vi "User Event Driver.vi"(11 "error in":errorcluster, 13 "LV2 Operation":T1) -> (4 "Stop":refnum<user-event>, 15 "error out":errorcluster)   [LabVIEW 2021, in "Game of Life.lvlib" / "User Event.lvlib"]
uses:
  User Event.lvlib
  controls/User Event Operations.ctl
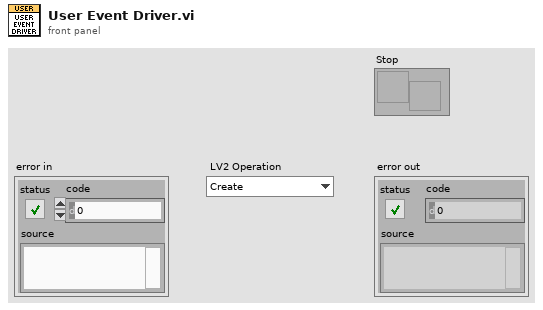
[diagram p1: front panel]
types:
  T1 = typedef "Game of Life.lvlib/User Event.lvlib/User Event Operations.ctl" = enum16{"Create", "Destroy", "Get Reference", "Generate"}
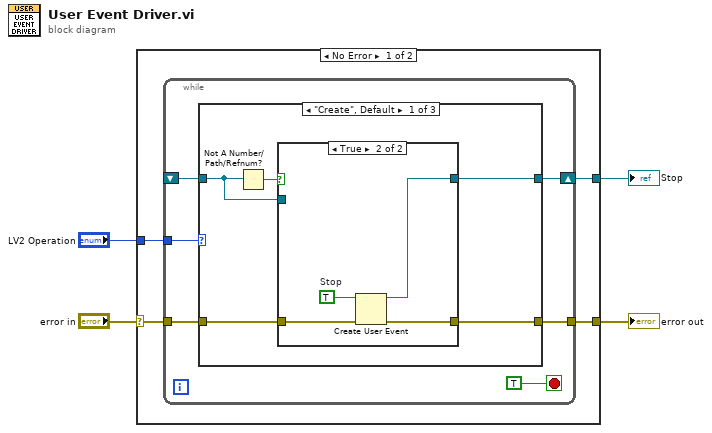
[diagram p0: block diagram]
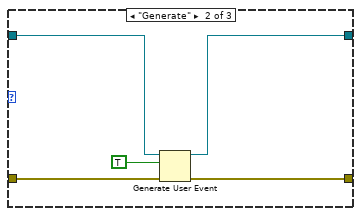
[diagram p3: hidden frame]
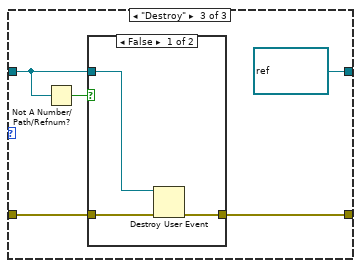
[diagram p4: hidden frame]
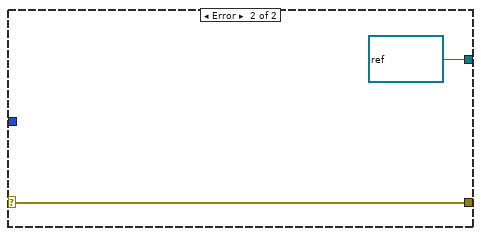
[diagram p6: hidden frame]
diagram:
  n1 = case shown="No Error" "error in" {
    selector: "error in" -> [w8 w41]
    tunnel: [w7 w41] -> w3
    tunnel: "LV2 Operation" -> [w6 _]
    tunnel: [w5 refnum<user-event> refnum ("Stop")] -> w1
    frame No Error {
      n2 = while {
        tunnel: w8 -> [w14]
        tunnel: [w13] -> w7
        tunnel: w6 -> [w11]
        shift-right: [w10] -> w5
        shift-left: _ -> [w9]
        stop <- TRUE stop-if-true
        n3 = case shown="\"Create\", Default" w11 {
          tunnel: [w18 w29 w34] -> w13
          tunnel: w14 -> [w19 w30 w35]
          tunnel: w9 -> [w16 w28 w32]
          tunnel: [w15 w26 refnum<user-event> refnum ("Stop")] -> w10
          frame "Create", Default {
            n4 = Not A Number/Path/Refnum?(number/path/refnum=w16) -> (NaN/Path/Refnum?=w17:bool)
            n5 = case shown="True" w17 {
              tunnel: w19 -> [w21 w25]
              tunnel: [w21 w24] -> w18
              tunnel: w16 -> [w20 _]
              tunnel: [w20 w22] -> w15
              frame False {
              }
              frame True {
                w23 = TRUE  # Stop
                n6 = Create User Event(user event datatype=w23, error in=w25) -> (user event=w22:refnum<user-event>, error out=w24:errorcluster)
              }
            }
          }
          frame "Generate" {
            n7 = Generate User Event(user event=w28, event data cluster=TRUE ("event data"), error in=w30) -> (user event out=w26:refnum<user-event>, error out=w29:errorcluster)  [unwired: 1 in]
          }
          frame "Destroy" {
            n8 = Not A Number/Path/Refnum?(number/path/refnum=w32) -> (NaN/Path/Refnum?=w33:bool)
            n9 = case shown="False" w33 {
              tunnel: w35 -> [w37 w39]
              tunnel: [w36 w39] -> w34
              tunnel: w32 -> [w38 _]
              frame False {
                n10 = Destroy User Event(user event=w38, error in=w37) -> (error out=w36:errorcluster)
              }
              frame True {
              }
            }
          }
        }
      }
    }
    frame Error {
    }
  }
  "error out" <- w3
  "Stop" <- w1
